vi "shag_start — 2.vi"() -> ()   [LabVIEW 2016]
uses:
  <vilib>/Instr/_visa.llb/VISA Configure Serial Port (Instr).vi
panel:
  in  "stop":bool
  out "положение в мин2":i32
  out "положение в мин 1":i32
  in  "?":T1(tab)
  in  "Минуты":i32 min=-600 max=11400
  in  "Задать текущее положение нулевым":bool
  out "положение шд":i32(knob) scale=-10.0..190.0
  in  "Вращение по градусам +":bool
  in  "Вращение по градусам -":bool
  out "текущее положение":string
  in  "Stop двигатель":bool
  in  "Установка минут":bool
  out "положение в минутах 1":string
  in  "Установка минут 2":bool
  in  "Задать текущее положение нулевым 2":bool
  in  "Вернуться в нулевое положение 2":bool
  in  "Вращение по градусам -  2":bool
  in  "Вращение по градусам +  2":bool
  in  "Stop двигатель 2":bool
  in  "Минуты 2":i32 min=-600 max=11400
  out "текущее положение 2":string
  out "положение шд 2":i32(knob) scale=-10.0..190.0
  out "положение в минутах 2":string
  in  "Блокировать\nРенгеновскую трубку":bool
  in  "Вернуться в нулевое положение":bool
  in  "Блокировать зеркало №1":bool
  in  "Выберете COM порт":refnum<visa-resource-name>="COM1"
  in  "Скорость обмена данными":u32(ring)=19200 items=["9600"=9600, "19200"=19200, "38400"=38400, "57600"=57600]
  in  "Число бит на символ":u16=8 min=5 max=8 step=1
  in  "Контроль чётности":enum16{"None", "Odd", "Even", "Mark", "Space"}(ring)
  in  "Стоповый бит":u16(ring)=10 items=["1.0"=10, "1.5"=15, "2.0"=20]
  in  "Контроль переполнения":u16(ring) items=["None"=0, "XON/XOFF"=1, "RTS/CTS"=2, "DTR/DSR"=4]
  # "1 - адресс 1 двигателя\n2 - адресс 2 двигателя\n$0MV\\01+   - запуск всех двигателей в положительном направлении \n$0MS\\00   - остановка всех двигателей\n$0MJ\\04+\\00\\00\\01   - 1 шаг всех двигателей\n$0SS\\01\\10   - скорость 10 для всех двигателей"
  # "Зеркало №1:"
  # "Положение:"
  # "Ренгеновская трубка №2:"
  # "Положение ренгеновской трубк:"
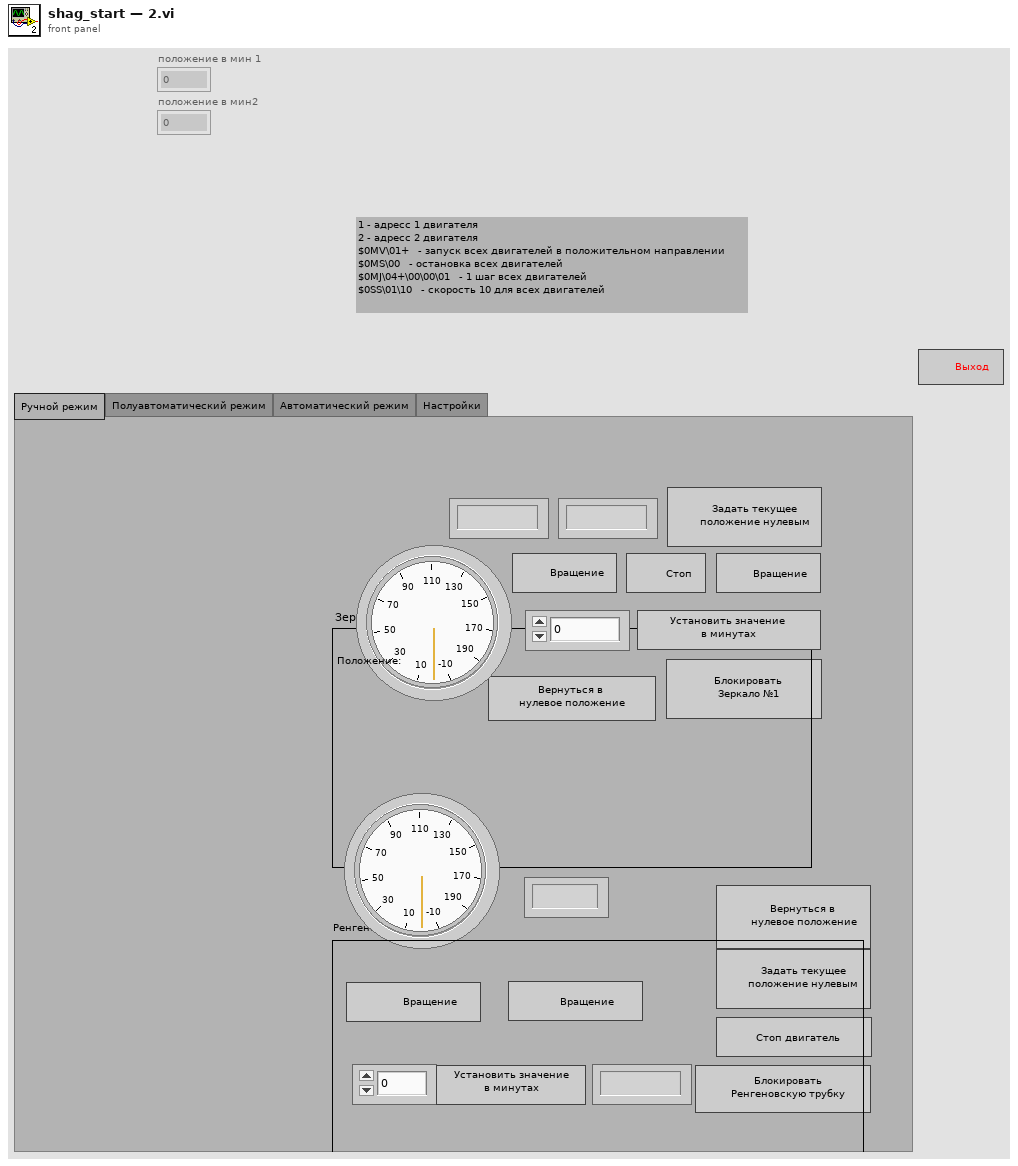
[diagram p1: front panel]
types:
  T1 = enum32{"Ручной режим", "Полуавтоматический режим", "Автоматический режим", "Настройки"}
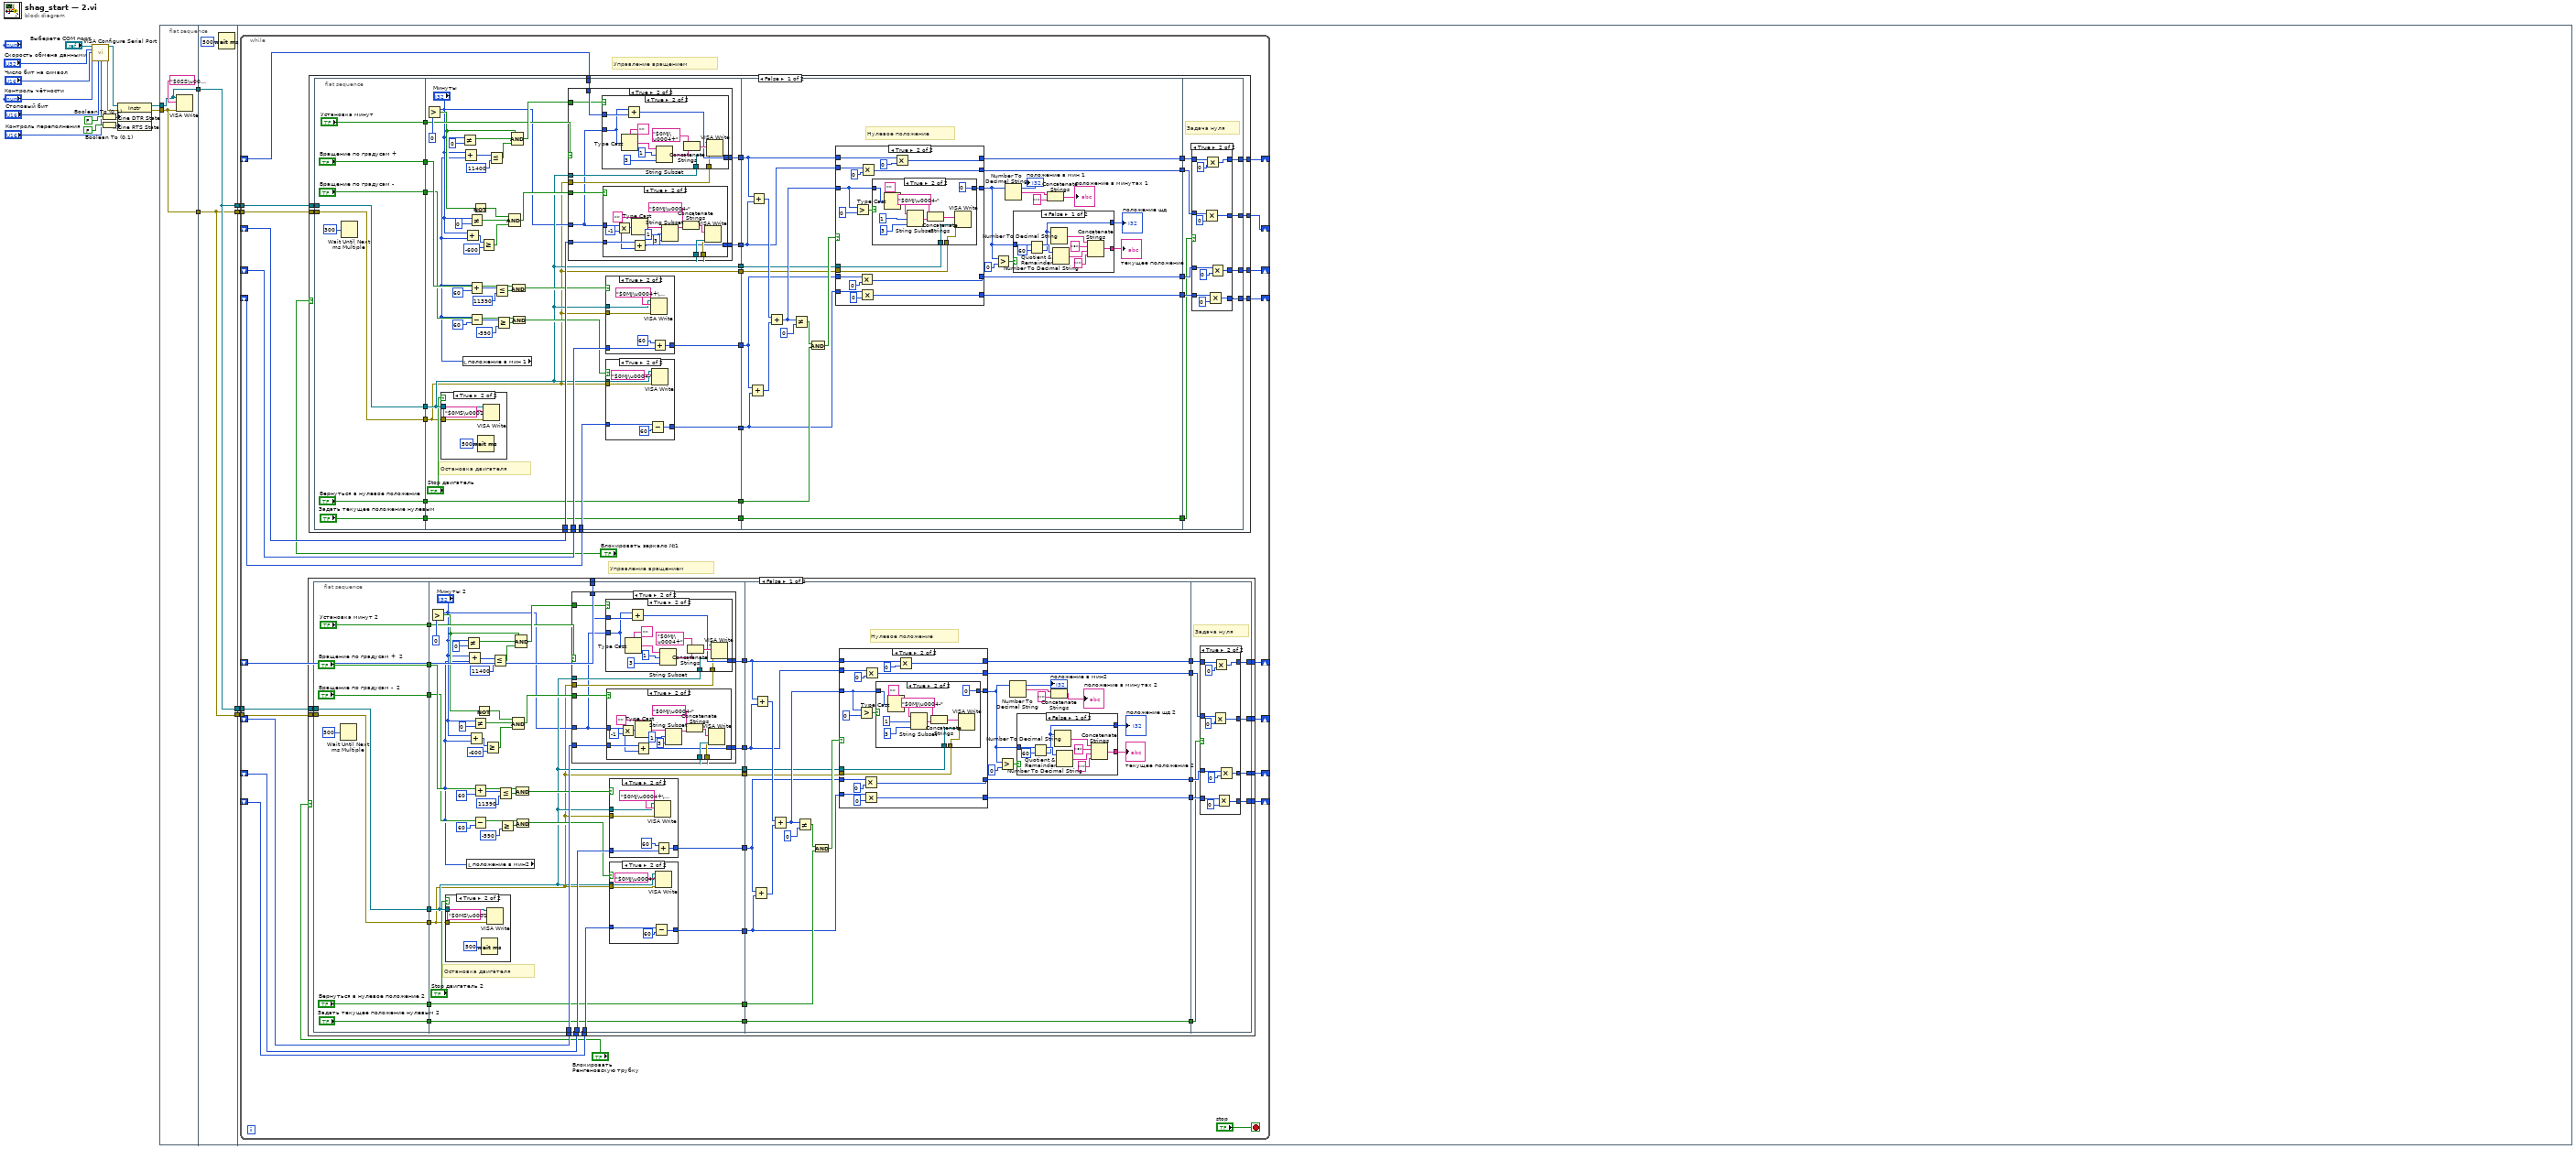
[diagram p0: block diagram]
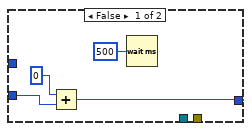
[diagram p3: hidden frame]
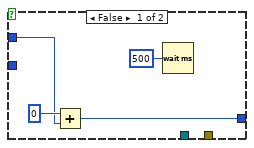
[diagram p4: hidden frame]
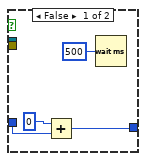
[diagram p6: hidden frame]
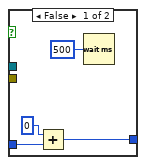
[diagram p7: hidden frame]
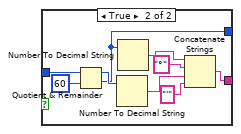
[diagram p8: hidden frame]
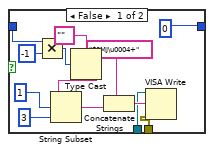
[diagram p10: hidden frame]
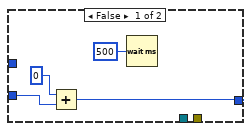
[diagram p14: hidden frame]
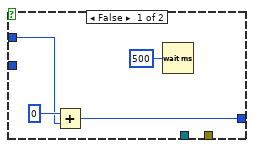
[diagram p15: hidden frame]
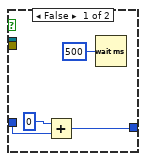
[diagram p17: hidden frame]
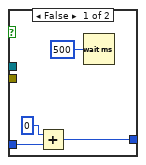
[diagram p18: hidden frame]
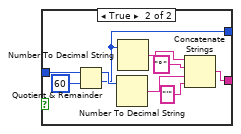
[diagram p19: hidden frame]
diagram:
  n1 = call-poly "VISA Configure Serial Port"("VISA resource name"="Выберете COM порт", "baud rate (9600)"="Скорость обмена данными", "data bits (8)"="Число бит на символ", "parity (0:none)"="Контроль чётности", "stop bits (10: 1 bit)"="Стоповый бит", "flow control (0:none)"="Контроль переполнения") -> ("VISA resource name out"=w18:refnum<visa-resource-name>, "error out"=w17:errorcluster)  [unwired: 8 in]
  n2 = Boolean To (0,1)(Boolean=FALSE ("DTR Write")) -> (0, 1=w19:i16)
  n3 = Boolean To (0,1)(Boolean=FALSE ("DTR Write")) -> (0, 1=w20:i16)
  n4 = property class="Instr"(reference=w18, error in=w17, "Serial Settings:Modem Line Settings:Line DTR State"=w19, "Serial Settings:Modem Line Settings:Line RTS State"=w20) -> (reference out=w16:refnum<visa-resource-name>, error out=w15:errorcluster)
  n5 = flat-sequence {
    tunnel: w16 -> [w22]
    tunnel: w15 -> [w21]
    tunnel: [w22] -> w13
    tunnel: [w21] -> w12
    tunnel: [w25] -> w14
    tunnel: w13 -> [w25]
    tunnel: w12 -> [w24]
    tunnel: [w24] -> w11
    tunnel: [w25] -> w2
    tunnel: [w24] -> w1
    tunnel: w14 -> [w30]
    tunnel: w11 -> [w29]
    tunnel: w2 -> [w28]
    tunnel: w1 -> [w27]
    frame #0 {
      n6 = VISA Write(VISA resource name=w22, write buffer="$0SS\u0001\u0010", error in (no error)=w21) -> ()  [unwired: 3 out]
    }
    frame #1 {
      n7 = Wait (ms)(milliseconds to wait=u32 500) -> ()  [unwired: 1 out]
    }
    frame #2 {
      n8 = while {
        tunnel: w30 -> [w51]
        tunnel: w29 -> [w50]
        shift-right: [w52] -> _
        shift-left: _ -> [w44]
        shift-right: [w49] -> _
        shift-left: _ -> [w45]
        shift-right: [w48] -> _
        shift-left: _ -> [w46]
        shift-right: [w47] -> _
        shift-left: _ -> [w43]
        tunnel: w28 -> [w41]
        tunnel: w27 -> [w40]
        shift-right: [w38] -> _
        shift-left: _ -> [w39]
        shift-right: [w34] -> _
        shift-left: _ -> [w37]
        shift-right: [w33] -> _
        shift-left: _ -> [w36]
        shift-right: [w32] -> _
        shift-left: _ -> [w35]
        stop <- "stop" stop-if-true
        # "Управление вращением"
        # "Управление вращением"
        n9 = case shown="False" "Блокировать\nРенгеновскую трубку" {
          tunnel: [w63 w323] -> w38
          tunnel: w41 -> [w62 _]
          tunnel: w40 -> [w61 _]
          tunnel: [w60 w322] -> w34
          tunnel: [w59 w321] -> w33
          tunnel: [w58 w320] -> w32
          tunnel: w36 -> [w57 w321]
          tunnel: w37 -> [w56 w322]
          tunnel: w39 -> [w55 w323]
          tunnel: w35 -> [w54 w320]
          frame False {
            n10 = flat-sequence {
              tunnel: w61 -> [w90]
              tunnel: w62 -> [w91]
              tunnel: [w91] -> w83
              tunnel: [w90] -> w82
              tunnel: ["Вращение по градусам +  2"] -> w81
              tunnel: ["Вращение по градусам -  2"] -> w80
              tunnel: ["Вернуться в нулевое положение 2"] -> w79
              tunnel: ["Задать текущее положение нулевым 2"] -> w78
              tunnel: ["Установка минут 2"] -> w77
              tunnel: w83 -> [w111]
              tunnel: w82 -> [w92]
              tunnel: [w134] -> w76
              tunnel: w55 -> [w131]
              tunnel: w56 -> [w133]
              tunnel: [w132] -> w75
              tunnel: w57 -> [w130]
              tunnel: w54 -> [w129]
              tunnel: w81 -> [w115]
              tunnel: w80 -> [w114]
              tunnel: [w128] -> w74
              tunnel: [w127] -> w73
              tunnel: [w112] -> w72
              tunnel: w79 -> [w112]
              tunnel: [w92] -> w71
              tunnel: [w111] -> w70
              tunnel: [w110] -> w69
              tunnel: w78 -> [w110]
              tunnel: w77 -> [w104]
              tunnel: w76 -> [w208]
              tunnel: w75 -> [w209]
              tunnel: [w229] -> w68
              tunnel: [w227] -> w67
              tunnel: w74 -> [w210]
              tunnel: w73 -> [w211]
              tunnel: [w217] -> w66
              tunnel: [w225] -> w65
              tunnel: w72 -> [w221]
              tunnel: w71 -> [w216]
              tunnel: w70 -> [w215]
              tunnel: w69 -> [w213]
              tunnel: [w213] -> w64
              tunnel: [w303] -> w63
              tunnel: [w300] -> w60
              tunnel: w68 -> [w302]
              tunnel: w67 -> [w301]
              tunnel: [w299] -> w59
              tunnel: [w298] -> w58
              tunnel: w66 -> [w297]
              tunnel: w65 -> [w296]
              tunnel: w64 -> [w295]
              frame #0 {
                n11 = Wait Until Next ms Multiple(millisecond multiple=u32 300) -> ()  [unwired: 1 out]
              }
              frame #1 {
                # "Остановка двигателя"
                n12 = Greater?(x="Минуты 2", y=0) -> (0:w102:bool)
                n13 = case shown="True" "Stop двигатель 2" {
                  tunnel: w111 -> [_ w181]
                  tunnel: w92 -> [_ w180]
                  frame False {
                  }
                  frame True {
                    n14 = Wait (ms)(milliseconds to wait=u32 500) -> ()  [unwired: 1 out]
                    n15 = VISA Write(VISA resource name=w181, write buffer="$0MS\u0001", error in (no error)=w180) -> ()  [unwired: 3 out]
                  }
                }
                n16 = Not Equal?(x="Минуты 2", y=0) -> (x != y?=w101:bool)
                n17 = local read "положение в мин2"() -> (w97:i32)
                n18 = Add(x="Минуты 2", y=w97) -> (x+y=w125:i32)
                n19 = Add(x="Минуты 2", y=w97) -> (x+y=w95:i32)
                n20 = Not Equal?(x="Минуты 2", y=0) -> (x != y?=w99:bool)
                n21 = Add(x=w97, y=60) -> (x+y=w120:i32)
                n22 = Subtract(x=w97, y=60) -> (x-y=w107:i32)
                n23 = Not(x=w102) -> (.not. x?=w103:bool)
                n24 = Greater Or Equal?(x=w95, y=-600) -> (x >= y?=w96:bool)
                n25 = Less Or Equal?(x=w125, y=11400) -> (x <= y?=w100:bool)
                n26 = Less Or Equal?(x=w120, y=11390) -> (x <= y?=w117:bool)
                n27 = Greater Or Equal?(x=w107, y=-590) -> (x >= y?=w108:bool)
                n28 = Compound Arithmetic op=AND(w103, w99, w96) -> (w121:bool)
                n29 = And(x=w115, y=w117) -> (x .and. y?=w116:bool)
                n30 = And(x=w114, y=w108) -> (x .and. y?=w113:bool)
                n31 = Compound Arithmetic op=AND(w102, w101, w100) -> (w123:bool)
                n32 = case shown="True" w104 {
                  tunnel: [w136 w145] -> w134
                  tunnel: w133 -> [w135 w144]
                  tunnel: [w135 w143] -> w132
                  tunnel: w131 -> [w136 w142]
                  tunnel: w123 -> [_ w141]
                  tunnel: w121 -> [_ w140]
                  tunnel: w92 -> [_ w139]
                  tunnel: w111 -> [_ w138]
                  tunnel: "Минуты 2" -> [_ w137]
                  frame False {
                  }
                  frame True {
                    n33 = case shown="True" w141 {
                      tunnel: [w166 w172] -> w145
                      tunnel: w142 -> [w165 w171]
                      tunnel: w139 -> [_ w170]
                      tunnel: w138 -> [_ w169]
                      tunnel: w137 -> [_ w168]
                      frame False {
                        n34 = Add(x=0, y=w165) -> (x+y=w166:i32)
                        n35 = Wait (ms)(milliseconds to wait=u32 500) -> ()  [unwired: 1 out]
                      }
                      frame True {
                        n36 = Type Cast(type="", x=w168) -> (*(type *) &x=w175:string)
                        n37 = Add(x=w168, y=w171) -> (x+y=w172:i32)
                        n38 = String Subset(string=w175, offset (0)=1, length (rest)=3 ("length (rest)")) -> (substring=w174:string)
                        n39 = Concatenate Strings("$0MJ\u0004+" ("write buffer"), w174) -> (w178:string)
                        n40 = VISA Write(VISA resource name=w169, write buffer=w178, error in (no error)=w170) -> ()  [unwired: 3 out]
                      }
                    }
                    n41 = case shown="True" w140 {
                      tunnel: [w148 w154] -> w143
                      tunnel: w144 -> [w147 w153]
                      tunnel: w138 -> [_ w156]
                      tunnel: w139 -> [_ w155]
                      tunnel: w137 -> [_ w150]
                      frame False {
                        n42 = Add(x=0, y=w147) -> (x+y=w148:i32)
                        n43 = Wait (ms)(milliseconds to wait=u32 500) -> ()  [unwired: 1 out]
                      }
                      frame True {
                        n44 = Multiply(x=w150, y=-1) -> (x*y=w152:i32)
                        n45 = Type Cast(type="", x=w152) -> (*(type *) &x=w159:string)
                        n46 = Add(x=w153, y=w150) -> (x+y=w154:i32)
                        n47 = String Subset(string=w159, offset (0)=1, length (rest)=3 ("length (rest)")) -> (substring=w158:string)
                        n48 = Concatenate Strings("$0MJ\u0004-" ("write buffer"), w158) -> (w162:string)
                        n49 = VISA Write(VISA resource name=w156, write buffer=w162, error in (no error)=w155) -> ()  [unwired: 3 out]
                      }
                    }
                  }
                }
                n50 = case shown="True" w116 {
                  tunnel: [w196 w203] -> w128
                  tunnel: w130 -> [w195 w198]
                  tunnel: w111 -> [_ w199]
                  tunnel: w92 -> [_ w200]
                  frame False {
                    n51 = Add(x=0, y=w195) -> (x+y=w196:i32)
                    n52 = Wait (ms)(milliseconds to wait=u32 500) -> ()  [unwired: 1 out]
                  }
                  frame True {
                    n53 = VISA Write(VISA resource name=w199, write buffer="$0MJ\u0004+\u0000\u0000<", error in (no error)=w200) -> ()  [unwired: 3 out]
                    n54 = Add(x=60, y=w198) -> (x+y=w203:i32)
                  }
                }
                n55 = case shown="True" w113 {
                  tunnel: [w186 w189] -> w127
                  tunnel: w129 -> [w185 w188]
                  tunnel: w111 -> [_ w192]
                  tunnel: w92 -> [_ w191]
                  frame False {
                    n56 = Add(x=0, y=w185) -> (x+y=w186:i32)
                    n57 = Wait (ms)(milliseconds to wait=u32 500) -> ()  [unwired: 1 out]
                  }
                  frame True {
                    n58 = Subtract(x=w188, y=60 ("x")) -> (x-y=w189:i32)
                    n59 = VISA Write(VISA resource name=w192, write buffer="$0MJ\u0004-\u0000\u0000<", error in (no error)=w191) -> ()  [unwired: 3 out]
                  }
                }
              }
              frame #2 {
                # "Нулевое положение"
                n60 = Add(x=w210, y=w211) -> (x+y=w222:i32)
                n61 = Add(x=w208, y=w209) -> (x+y=w226:i32)
                n62 = Add(x=w226, y=w222) -> (x+y=w219:i32)
                n63 = Not Equal?(x=w219, y=0 ("x")) -> (x != y?=w218:bool)
                n64 = And(x=w218, y=w221) -> (x .and. y?=w228:bool)
                n65 = case shown="True" w228 {
                  tunnel: [w250 w270] -> w205
                  tunnel: w208 -> [w252 w267]
                  tunnel: [w252 w266] -> w229
                  tunnel: [w251 w265] -> w227
                  tunnel: w219 -> [w250 w259]
                  tunnel: [w248 w261] -> w225
                  tunnel: [w249 w258] -> w217
                  tunnel: w209 -> [w251 w257]
                  tunnel: w216 -> [_ w256]
                  tunnel: w215 -> [_ w255]
                  tunnel: w210 -> [w249 w254]
                  tunnel: w211 -> [w248 w253]
                  frame False {
                  }
                  frame True {
                    n66 = Greater?(x=w259, y=0) -> (0:w260:bool)
                    n67 = Multiply(x=w254, y=0) -> (x*y=w258:i32)
                    n68 = Multiply(x=w253, y=0) -> (x*y=w261:i32)
                    n69 = Multiply(x=w257, y=0) -> (x*y=w265:i32)
                    n70 = case shown="True" w260 {
                      tunnel: w259 -> [w275 w288]
                      tunnel: [0 0] -> w270
                      tunnel: w255 -> [w272 w285]
                      tunnel: w256 -> [w271 w284]
                      frame False {
                        n71 = Multiply(x=w275, y=-1) -> (x*y=w273:i32)
                        n72 = Type Cast(type="", x=w273) -> (*(type *) &x=w279:string)
                        n73 = String Subset(string=w279, offset (0)=1, length (rest)=3 ("length (rest)")) -> (substring=w278:string)
                        n74 = Concatenate Strings("$0MJ\u0004+" ("write buffer"), w278) -> (w282:string)
                        n75 = VISA Write(VISA resource name=w272, write buffer=w282, error in (no error)=w271) -> ()  [unwired: 3 out]
                      }
                      frame True {
                        n76 = Type Cast(type="", x=w288) -> (*(type *) &x=w291:string)
                        n77 = String Subset(string=w291, offset (0)=1, length (rest)=3 ("length (rest)")) -> (substring=w290:string)
                        n78 = Concatenate Strings("$0MJ\u0004-" ("write buffer"), w290) -> (w286:string)
                        n79 = VISA Write(VISA resource name=w285, write buffer=w286, error in (no error)=w284) -> ()  [unwired: 3 out]
                      }
                    }
                    n80 = Multiply(x=w267, y=0) -> (x*y=w266:i32)
                  }
                }
                "положение в мин2" <- w205
                n81 = Greater?(x=w205, y=0) -> (0:w224:bool)
                n82 = Number To Decimal String(number=w205) -> (decimal integer string=w206:string)  [unwired: 1 in]
                n83 = case shown="False" w224 {
                  tunnel: w205 -> [w237 w247]
                  tunnel: [w234 w241] -> w214
                  tunnel: [w230 w239] -> w212
                  frame False {
                    n84 = Quotient & Remainder(x=w237, y=60) -> (x-y*floor(x/y)=w233:i32, floor(x/y)=w230:i32)
                    n85 = Number To Decimal String(number=w230) -> (decimal integer string=w231:string)  [unwired: 1 in]
                    n86 = Number To Decimal String(number=w233) -> (decimal integer string=w232:string)  [unwired: 1 in]
                    n87 = Concatenate Strings(w231, "°" ("string"), w232, "'" ("string")) -> (w234:string)
                  }
                  frame True {
                    n88 = Quotient & Remainder(x=w247, y=60) -> (x-y*floor(x/y)=w240:i32, floor(x/y)=w239:i32)
                    n89 = Number To Decimal String(number=w240) -> (decimal integer string=w242:string)  [unwired: 1 in]
                    n90 = Number To Decimal String(number=w239) -> (decimal integer string=w243:string)  [unwired: 1 in]
                    n91 = Concatenate Strings(w243, "°" ("string"), w242, "'" ("string")) -> (w241:string)
                  }
                }
                "положение шд 2" <- w212
                "текущее положение 2" <- w214
                n92 = Concatenate Strings(w206, "'" ("string")) -> (→"положение в минутах 2":string)
              }
              frame #3 {
                # "Задача нуля"
                n93 = case shown="True" w295 {
                  tunnel: [w307 w318] -> w303
                  tunnel: w302 -> [w307 w319]
                  tunnel: w301 -> [w306 w315]
                  tunnel: [w306 w314] -> w300
                  tunnel: [w305 w311] -> w299
                  tunnel: [w304 w310] -> w298
                  tunnel: w297 -> [w305 w309]
                  tunnel: w296 -> [w304 w308]
                  frame False {
                  }
                  frame True {
                    n94 = Multiply(x=w315, y=0) -> (x*y=w314:i32)
                    n95 = Multiply(x=w319, y=0) -> (x*y=w318:i32)
                    n96 = Multiply(x=w308, y=0) -> (x*y=w310:i32)
                    n97 = Multiply(x=w309, y=0) -> (x*y=w311:i32)
                  }
                }
              }
            }
          }
          frame True {
          }
        }
        n98 = case shown="False" "Блокировать зеркало №1" {
          tunnel: [w333 w593] -> w52
          tunnel: w51 -> [w332 _]
          tunnel: w50 -> [w331 _]
          tunnel: [w330 w592] -> w49
          tunnel: [w329 w591] -> w48
          tunnel: [w328 w590] -> w47
          tunnel: w46 -> [w327 w591]
          tunnel: w45 -> [w326 w592]
          tunnel: w44 -> [w325 w593]
          tunnel: w43 -> [w324 w590]
          frame False {
            n99 = flat-sequence {
              tunnel: w331 -> [w360]
              tunnel: w332 -> [w361]
              tunnel: [w361] -> w353
              tunnel: [w360] -> w352
              tunnel: ["Вращение по градусам +"] -> w351
              tunnel: ["Вращение по градусам -"] -> w350
              tunnel: ["Вернуться в нулевое положение"] -> w349
              tunnel: ["Задать текущее положение нулевым"] -> w348
              tunnel: ["Установка минут"] -> w347
              tunnel: w353 -> [w381]
              tunnel: w352 -> [w362]
              tunnel: [w404] -> w346
              tunnel: w325 -> [w401]
              tunnel: w326 -> [w403]
              tunnel: [w402] -> w345
              tunnel: w327 -> [w400]
              tunnel: w324 -> [w399]
              tunnel: w351 -> [w385]
              tunnel: w350 -> [w384]
              tunnel: [w398] -> w344
              tunnel: [w397] -> w343
              tunnel: [w382] -> w342
              tunnel: w349 -> [w382]
              tunnel: [w362] -> w341
              tunnel: [w381] -> w340
              tunnel: [w380] -> w339
              tunnel: w348 -> [w380]
              tunnel: w347 -> [w374]
              tunnel: w346 -> [w478]
              tunnel: w345 -> [w479]
              tunnel: [w499] -> w338
              tunnel: [w497] -> w337
              tunnel: w344 -> [w480]
              tunnel: w343 -> [w481]
              tunnel: [w487] -> w336
              tunnel: [w495] -> w335
              tunnel: w342 -> [w491]
              tunnel: w341 -> [w486]
              tunnel: w340 -> [w485]
              tunnel: w339 -> [w483]
              tunnel: [w483] -> w334
              tunnel: [w573] -> w333
              tunnel: [w570] -> w330
              tunnel: w338 -> [w572]
              tunnel: w337 -> [w571]
              tunnel: [w569] -> w329
              tunnel: [w568] -> w328
              tunnel: w336 -> [w567]
              tunnel: w335 -> [w566]
              tunnel: w334 -> [w565]
              frame #0 {
                n100 = Wait Until Next ms Multiple(millisecond multiple=u32 300) -> ()  [unwired: 1 out]
              }
              frame #1 {
                # "Остановка двигателя"
                n101 = Greater?(x="Минуты", y=0) -> (0:w372:bool)
                n102 = case shown="True" "Stop двигатель" {
                  tunnel: w381 -> [_ w451]
                  tunnel: w362 -> [_ w450]
                  frame False {
                  }
                  frame True {
                    n103 = Wait (ms)(milliseconds to wait=u32 500) -> ()  [unwired: 1 out]
                    n104 = VISA Write(VISA resource name=w451, write buffer="$0MS\u0001", error in (no error)=w450) -> ()  [unwired: 3 out]
                  }
                }
                n105 = Not Equal?(x="Минуты", y=0) -> (x != y?=w371:bool)
                n106 = local read "положение в мин 1"() -> (w367:i32)
                n107 = Add(x="Минуты", y=w367) -> (x+y=w395:i32)
                n108 = Add(x="Минуты", y=w367) -> (x+y=w365:i32)
                n109 = Not Equal?(x="Минуты", y=0) -> (x != y?=w369:bool)
                n110 = Add(x=w367, y=60) -> (x+y=w390:i32)
                n111 = Subtract(x=w367, y=60) -> (x-y=w377:i32)
                n112 = Not(x=w372) -> (.not. x?=w373:bool)
                n113 = Greater Or Equal?(x=w365, y=-600) -> (x >= y?=w366:bool)
                n114 = Less Or Equal?(x=w395, y=11400) -> (x <= y?=w370:bool)
                n115 = Less Or Equal?(x=w390, y=11390) -> (x <= y?=w387:bool)
                n116 = Greater Or Equal?(x=w377, y=-590) -> (x >= y?=w378:bool)
                n117 = Compound Arithmetic op=AND(w373, w369, w366) -> (w391:bool)
                n118 = And(x=w385, y=w387) -> (x .and. y?=w386:bool)
                n119 = And(x=w384, y=w378) -> (x .and. y?=w383:bool)
                n120 = Compound Arithmetic op=AND(w372, w371, w370) -> (w393:bool)
                n121 = case shown="True" w374 {
                  tunnel: [w406 w415] -> w404
                  tunnel: w403 -> [w405 w414]
                  tunnel: [w405 w413] -> w402
                  tunnel: w401 -> [w406 w412]
                  tunnel: w393 -> [_ w411]
                  tunnel: w391 -> [_ w410]
                  tunnel: w362 -> [_ w409]
                  tunnel: w381 -> [_ w408]
                  tunnel: "Минуты" -> [_ w407]
                  frame False {
                  }
                  frame True {
                    n122 = case shown="True" w411 {
                      tunnel: [w436 w442] -> w415
                      tunnel: w412 -> [w435 w441]
                      tunnel: w409 -> [_ w440]
                      tunnel: w408 -> [_ w439]
                      tunnel: w407 -> [_ w438]
                      frame False {
                        n123 = Add(x=0, y=w435) -> (x+y=w436:i32)
                        n124 = Wait (ms)(milliseconds to wait=u32 500) -> ()  [unwired: 1 out]
                      }
                      frame True {
                        n125 = Type Cast(type="", x=w438) -> (*(type *) &x=w445:string)
                        n126 = Add(x=w438, y=w441) -> (x+y=w442:i32)
                        n127 = String Subset(string=w445, offset (0)=1, length (rest)=3 ("length (rest)")) -> (substring=w444:string)
                        n128 = Concatenate Strings("$0MJ\u0004+" ("write buffer"), w444) -> (w448:string)
                        n129 = VISA Write(VISA resource name=w439, write buffer=w448, error in (no error)=w440) -> ()  [unwired: 3 out]
                      }
                    }
                    n130 = case shown="True" w410 {
                      tunnel: [w418 w424] -> w413
                      tunnel: w414 -> [w417 w423]
                      tunnel: w408 -> [_ w426]
                      tunnel: w409 -> [_ w425]
                      tunnel: w407 -> [_ w420]
                      frame False {
                        n131 = Add(x=0, y=w417) -> (x+y=w418:i32)
                        n132 = Wait (ms)(milliseconds to wait=u32 500) -> ()  [unwired: 1 out]
                      }
                      frame True {
                        n133 = Multiply(x=w420, y=-1) -> (x*y=w422:i32)
                        n134 = Type Cast(type="", x=w422) -> (*(type *) &x=w429:string)
                        n135 = Add(x=w423, y=w420) -> (x+y=w424:i32)
                        n136 = String Subset(string=w429, offset (0)=1, length (rest)=3 ("length (rest)")) -> (substring=w428:string)
                        n137 = Concatenate Strings("$0MJ\u0004-" ("write buffer"), w428) -> (w432:string)
                        n138 = VISA Write(VISA resource name=w426, write buffer=w432, error in (no error)=w425) -> ()  [unwired: 3 out]
                      }
                    }
                  }
                }
                n139 = case shown="True" w386 {
                  tunnel: [w466 w473] -> w398
                  tunnel: w400 -> [w465 w468]
                  tunnel: w381 -> [_ w469]
                  tunnel: w362 -> [_ w470]
                  frame False {
                    n140 = Add(x=0, y=w465) -> (x+y=w466:i32)
                    n141 = Wait (ms)(milliseconds to wait=u32 500) -> ()  [unwired: 1 out]
                  }
                  frame True {
                    n142 = VISA Write(VISA resource name=w469, write buffer="$0MJ\u0004+\u0000\u0000<", error in (no error)=w470) -> ()  [unwired: 3 out]
                    n143 = Add(x=60, y=w468) -> (x+y=w473:i32)
                  }
                }
                n144 = case shown="True" w383 {
                  tunnel: [w456 w459] -> w397
                  tunnel: w399 -> [w455 w458]
                  tunnel: w381 -> [_ w462]
                  tunnel: w362 -> [_ w461]
                  frame False {
                    n145 = Add(x=0, y=w455) -> (x+y=w456:i32)
                    n146 = Wait (ms)(milliseconds to wait=u32 500) -> ()  [unwired: 1 out]
                  }
                  frame True {
                    n147 = Subtract(x=w458, y=60 ("x")) -> (x-y=w459:i32)
                    n148 = VISA Write(VISA resource name=w462, write buffer="$0MJ\u0004-\u0000\u0000<", error in (no error)=w461) -> ()  [unwired: 3 out]
                  }
                }
              }
              frame #2 {
                # "Нулевое положение"
                n149 = Add(x=w480, y=w481) -> (x+y=w492:i32)
                n150 = Add(x=w478, y=w479) -> (x+y=w496:i32)
                n151 = Add(x=w496, y=w492) -> (x+y=w489:i32)
                n152 = Not Equal?(x=w489, y=0 ("x")) -> (x != y?=w488:bool)
                n153 = And(x=w488, y=w491) -> (x .and. y?=w498:bool)
                n154 = case shown="True" w498 {
                  tunnel: [w520 w540] -> w477
                  tunnel: w478 -> [w522 w537]
                  tunnel: [w522 w536] -> w499
                  tunnel: [w521 w535] -> w497
                  tunnel: w489 -> [w520 w529]
                  tunnel: [w518 w531] -> w495
                  tunnel: [w519 w528] -> w487
                  tunnel: w479 -> [w521 w527]
                  tunnel: w486 -> [_ w526]
                  tunnel: w485 -> [_ w525]
                  tunnel: w480 -> [w519 w524]
                  tunnel: w481 -> [w518 w523]
                  frame False {
                  }
                  frame True {
                    n155 = Greater?(x=w529, y=0) -> (0:w530:bool)
                    n156 = Multiply(x=w524, y=0) -> (x*y=w528:i32)
                    n157 = Multiply(x=w523, y=0) -> (x*y=w531:i32)
                    n158 = Multiply(x=w527, y=0) -> (x*y=w535:i32)
                    n159 = case shown="True" w530 {
                      tunnel: w529 -> [w545 w558]
                      tunnel: [0 0] -> w540
                      tunnel: w525 -> [w542 w555]
                      tunnel: w526 -> [w541 w554]
                      frame False {
                        n160 = Multiply(x=w545, y=-1) -> (x*y=w543:i32)
                        n161 = Type Cast(type="", x=w543) -> (*(type *) &x=w549:string)
                        n162 = String Subset(string=w549, offset (0)=1, length (rest)=3 ("length (rest)")) -> (substring=w548:string)
                        n163 = Concatenate Strings("$0MJ\u0004+" ("write buffer"), w548) -> (w552:string)
                        n164 = VISA Write(VISA resource name=w542, write buffer=w552, error in (no error)=w541) -> ()  [unwired: 3 out]
                      }
                      frame True {
                        n165 = Type Cast(type="", x=w558) -> (*(type *) &x=w561:string)
                        n166 = String Subset(string=w561, offset (0)=1, length (rest)=3 ("length (rest)")) -> (substring=w560:string)
                        n167 = Concatenate Strings("$0MJ\u0004-" ("write buffer"), w560) -> (w556:string)
                        n168 = VISA Write(VISA resource name=w555, write buffer=w556, error in (no error)=w554) -> ()  [unwired: 3 out]
                      }
                    }
                    n169 = Multiply(x=w537, y=0) -> (x*y=w536:i32)
                  }
                }
                "положение в мин 1" <- w477
                n170 = Greater?(x=w477, y=0) -> (0:w494:bool)
                n171 = Number To Decimal String(number=w477) -> (decimal integer string=w475:string)  [unwired: 1 in]
                n172 = case shown="False" w494 {
                  tunnel: w477 -> [w507 w517]
                  tunnel: [w504 w511] -> w484
                  tunnel: [w500 w509] -> w482
                  frame False {
                    n173 = Quotient & Remainder(x=w507, y=60) -> (x-y*floor(x/y)=w503:i32, floor(x/y)=w500:i32)
                    n174 = Number To Decimal String(number=w500) -> (decimal integer string=w501:string)  [unwired: 1 in]
                    n175 = Number To Decimal String(number=w503) -> (decimal integer string=w502:string)  [unwired: 1 in]
                    n176 = Concatenate Strings(w501, "°" ("string"), w502, "'" ("string")) -> (w504:string)
                  }
                  frame True {
                    n177 = Quotient & Remainder(x=w517, y=60) -> (x-y*floor(x/y)=w510:i32, floor(x/y)=w509:i32)
                    n178 = Number To Decimal String(number=w510) -> (decimal integer string=w512:string)  [unwired: 1 in]
                    n179 = Number To Decimal String(number=w509) -> (decimal integer string=w513:string)  [unwired: 1 in]
                    n180 = Concatenate Strings(w513, "°" ("string"), w512, "'" ("string")) -> (w511:string)
                  }
                }
                "положение шд" <- w482
                "текущее положение" <- w484
                n181 = Concatenate Strings(w475, "'" ("string")) -> (→"положение в минутах 1":string)
              }
              frame #3 {
                # "Задача нуля"
                n182 = case shown="True" w565 {
                  tunnel: [w577 w588] -> w573
                  tunnel: w572 -> [w577 w589]
                  tunnel: w571 -> [w576 w585]
                  tunnel: [w576 w584] -> w570
                  tunnel: [w575 w581] -> w569
                  tunnel: [w574 w580] -> w568
                  tunnel: w567 -> [w575 w579]
                  tunnel: w566 -> [w574 w578]
                  frame False {
                  }
                  frame True {
                    n183 = Multiply(x=w585, y=0) -> (x*y=w584:i32)
                    n184 = Multiply(x=w589, y=0) -> (x*y=w588:i32)
                    n185 = Multiply(x=w578, y=0) -> (x*y=w580:i32)
                    n186 = Multiply(x=w579, y=0) -> (x*y=w581:i32)
                  }
                }
              }
            }
          }
          frame True {
          }
        }
      }
    }
  }
